vi "Enqueue Update Panel Message.vi"(6 "Priority Message? (F)":bool, 8 "error in (no error)":errorcluster[](array[cluster]), 11 "Message Queue":refnum<queue>) -> (0 "error out":errorcluster[](array[cluster]), 3 "dup Message Queue":refnum<queue>)   [LabVIEW 2018, in "Message Queue.lvlib"]
doc: "For a regular message, enqueue the message. For a priority message, enqueue it at the front of the queue."
uses:
  Message Queue.lvlib
  Message Cluster.ctl
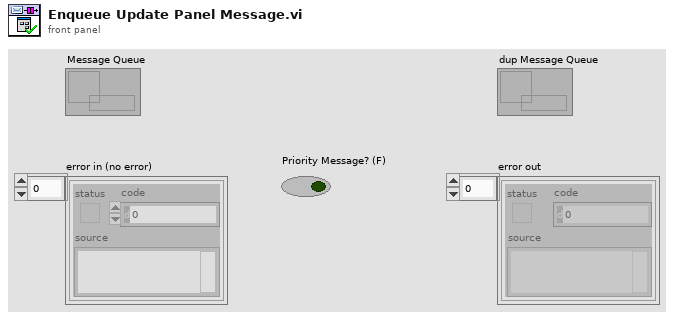
[diagram p1: front panel]
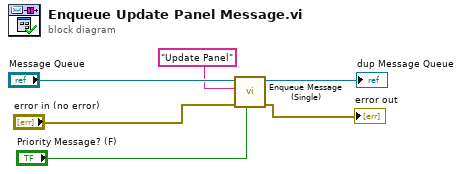
[diagram p0: block diagram]
diagram:
  n1 = call "Enqueue Message (Single).vi"("Priority Message? (F)"="Priority Message? (F)", "error in (no error)"="error in (no error)", "Message"="Update Panel", "Message Queue"="Message Queue") -> ("error out"=→"error out":errorcluster[], "dup Message Queue"=→"dup Message Queue":refnum<queue>)  [unwired: 6 in]
